vi "BlinkLight.vi"(1 "Blink Interval (ms)":u32=100) -> (0 "Blinked Output":bool)   [LabVIEW 2019]
doc: "This VI may be used to blink an indicator \"On\" and \"Off.\" While you can use it for other applications, there are no settings to safely control reinitialization etc. Therefore this VI should not be used for any safety-critical actuator outputs."
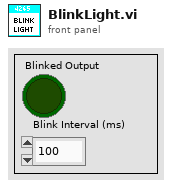
[diagram p1: front panel]
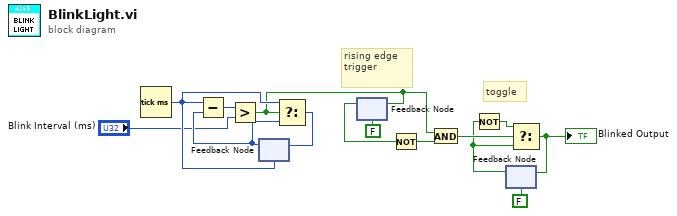
[diagram p0: block diagram]
diagram:
  # "toggle"
  # "rising edge\ntrigger"
  n1 = Tick Count (ms)() -> (millisecond timer value=w13:u32)
  n2 = feedback #1(w13) -> (w12:u32)
  n3 = Subtract(x=w13, y=w12) -> (x-y=w11:u32)
  n4 = Greater?(x=w11, y="Blink Interval (ms)") -> (0:w6:bool)
  n5 = Select(t=w13, s=w6, f=w12) -> (s? t:f=w14:u32)
  n6 = feedback-in #1(w14) -> ()
  n7 = feedback #2(FALSE ("Button")) -> (w7:bool)
  n8 = feedback-in #2(w6) -> ()
  n9 = Not(x=w7) -> (.not. x?=w9:bool)
  n10 = And(x=w6, y=w9) -> (x .and. y?=w5:bool)
  n11 = feedback #3(FALSE) -> (w3:bool)
  n12 = Not(x=w3) -> (.not. x?=w4:bool)
  n13 = Select(t=w4, s=w5, f=w3) -> (s? t:f=w2:bool)
  "Blinked Output" <- w2
  n14 = feedback-in #3(w2) -> ()
